vi "Syringe Freezer Interlock Configuration.vi"(8 "error in (no error)":errorcluster, 11 "cRIO-CO2 in":refnum<class "cRIO-CO2.lvclass">) -> (0 "error out":errorcluster, 2 "Interlock Chain":refnum<class "Interlock Chain.lvclass">, 3 "cRIO-CO2 out":refnum<class "cRIO-CO2.lvclass">)   [LabVIEW 2015, in "cRIO-Carbondioxide.lvlib" / "cRIO-CO2.lvlib" / "cRIO-CO2.lvclass"]
uses:
  cRIO-CO2.lvclass
  Interlocks/Interlock Chain/Interlock Chain.lvclass
  Interlocks/Interlock/Interlock.lvclass
  Interlocks/Interlock Bool/Interlock Bool.lvclass
  Interlocks/Interlock DBL/Range/Interlock Range.lvclass
  Interlocks/Interlock Bool/Interlock Bool.lvclass/Interlock Bool.ctl
  Interlocks/Interlock DBL/Range/Interlock Range.lvclass/Interlock Range.ctl
  Interlocks/Interlock Chain/Interlock Chain.lvclass/Interlock Chain.ctl
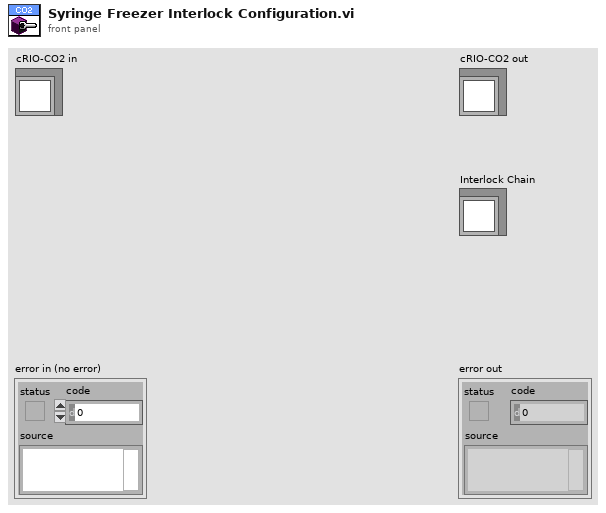
[diagram p1: front panel]
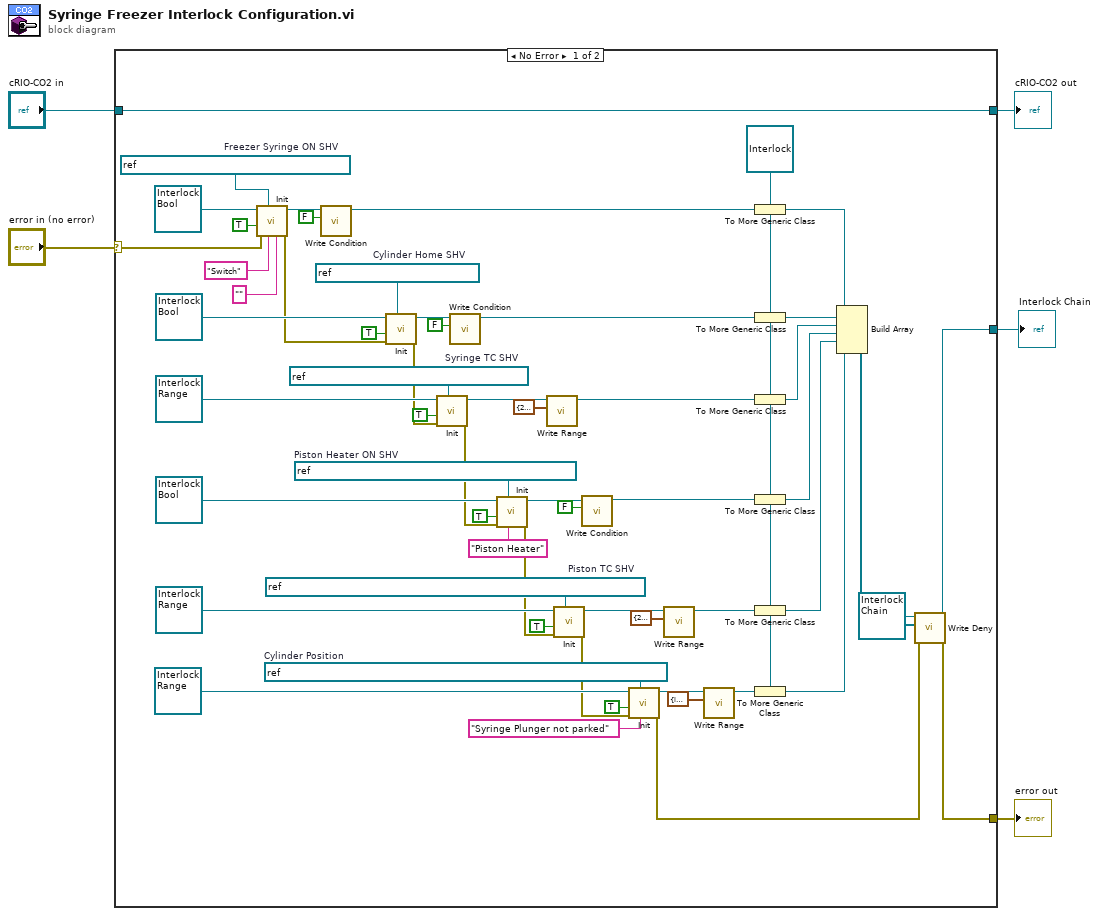
[diagram p0: block diagram]
diagram:
  n1 = case shown="No Error" "error in (no error)" {
    selector: "error in (no error)" -> [w30 w66]
    tunnel: [w25 w66] -> w4
    tunnel: [w64 w65] -> w2
    tunnel: "cRIO-CO2 in" -> [w64 w65]
    tunnel: [w22 _] -> w1
    frame No Error {
      w12 = refnum<k21> "ni.var.psp://crio-carbondioxide/AMS Gas SHV/Cylinder/Position"  # Cylinder Position
      w36 = refnum<k21> "ni.var.psp://crio-carbondioxide/AMS Gas SHV/Freezers/Freezer Syringe"  # Freezer Syringe ON SHV
      w41 = refnum<k21> "ni.var.psp://crio-carbondioxide/AMS Gas SHV/Gauges/Piston TC"  # Piston TC SHV
      w51 = refnum<k21> "ni.var.psp://crio-carbondioxide/AMS Gas SHV/Heaters/Piston Heater ON"  # Piston Heater ON SHV
      w55 = refnum<k21> "ni.var.psp://crio-carbondioxide/AMS Gas SHV/Gauges/Syringe TC"  # Syringe TC SHV
      w8 = refnum<class "Interlock.lvclass"> refnum ("Interlock.lvclass")
      w62 = refnum<k21> "ni.var.psp://crio-carbondioxide/AMS Gas SHV/Cylinder/Home"  # Cylinder Home SHV
      n2 = call-dynamic "Init.vi"("Interlock message (\" -> Interlock!\")"="" ("Interlock message (\" -> Interlock!\")"), "Name (SHV Name if empty)"="Switch", "SHV"=w36, "error in (no error)"=w30, "Stop Self on IL? (T)"=TRUE, "Interlock in"=refnum<class "Interlock Bool.lvclass"> refnum ("Interlock Bool.lvclass")) -> ("error out"=w31:errorcluster, "Interlock out"=w37:refnum<class "Interlock Bool.lvclass">)  [unwired: 4 in]
      n3 = call "Write Condition.vi"("Interlock Condition"=FALSE, "Interlock Bool in"=w37) -> ("Interlock Bool out"=w28:refnum<class "Interlock Bool.lvclass">)  [unwired: 8 in, 1 out]
      n4 = call-dynamic "Init.vi"("SHV"=w62, "error in (no error)"=w31, "Stop Self on IL? (T)"=TRUE, "Interlock in"=refnum<class "Interlock Bool.lvclass"> refnum ("Interlock Bool.lvclass")) -> ("error out"=w34:errorcluster, "Interlock out"=w61:refnum<class "Interlock Bool.lvclass">)  [unwired: 6 in]
      n5 = call-dynamic "Init.vi"("SHV"=w55, "error in (no error)"=w34, "Stop Self on IL? (T)"=TRUE, "Interlock in"=refnum<class "Interlock Range.lvclass"> refnum ("Interlock DBL.lvclass")) -> ("error out"=w33:errorcluster, "Interlock out"=w56:refnum<class "Interlock Range.lvclass">)  [unwired: 6 in]
      n6 = call "Write Condition.vi"("Interlock Condition"=FALSE, "Interlock Bool in"=w61) -> ("Interlock Bool out"=w59:refnum<class "Interlock Bool.lvclass">)  [unwired: 8 in, 1 out]
      n7 = call-dynamic "Init.vi"("Name (SHV Name if empty)"="Piston Heater", "SHV"=w51, "error in (no error)"=w33, "Stop Self on IL? (T)"=TRUE, "Interlock in"=refnum<class "Interlock Bool.lvclass"> refnum ("Interlock Bool.lvclass")) -> ("error out"=w32:errorcluster, "Interlock out"=w49:refnum<class "Interlock Bool.lvclass">)  [unwired: 5 in]
      n8 = call "Write Range.vi"("Range"=cluster{"Upper Limit":dbl, "Lower Limit":dbl} {"Upper Limit"=2000.0, "Lower Limit"=-200.0}, "Interlock Bool in"=w56) -> ("Interlock Bool out"=w53:refnum<class "Interlock Range.lvclass">)  [unwired: 8 in, 1 out]
      n9 = call-dynamic "Init.vi"("SHV"=w41, "error in (no error)"=w32, "Stop Self on IL? (T)"=TRUE, "Interlock in"=refnum<class "Interlock Range.lvclass"> refnum ("Interlock DBL.lvclass")) -> ("error out"=w15:errorcluster, "Interlock out"=w43:refnum<class "Interlock Range.lvclass">)  [unwired: 6 in]
      n10 = call "Write Condition.vi"("Interlock Condition"=FALSE, "Interlock Bool in"=w49) -> ("Interlock Bool out"=w47:refnum<class "Interlock Bool.lvclass">)  [unwired: 8 in, 1 out]
      n11 = call-dynamic "Init.vi"("Name (SHV Name if empty)"="Syringe Plunger not parked", "SHV"=w12, "error in (no error)"=w15, "Stop Self on IL? (T)"=TRUE, "Interlock in"=refnum<class "Interlock Range.lvclass"> refnum ("Interlock DBL.lvclass")) -> ("error out"=w14:errorcluster, "Interlock out"=w11:refnum<class "Interlock Range.lvclass">)  [unwired: 5 in]
      n12 = call "Write Range.vi"("Range"=cluster{"Upper Limit":dbl, "Lower Limit":dbl} {"Upper Limit"=2000.0, "Lower Limit"=20.0}, "Interlock Bool in"=w43) -> ("Interlock Bool out"=w40:refnum<class "Interlock Range.lvclass">)  [unwired: 8 in, 1 out]
      n13 = call "Write Range.vi"("Range"=cluster{"Upper Limit":dbl, "Lower Limit":dbl} {"Upper Limit"=inf, "Lower Limit"=95.0}, "Interlock Bool in"=w11) -> ("Interlock Bool out"=w9:refnum<class "Interlock Range.lvclass">)  [unwired: 8 in, 1 out]
      n14 = To More Generic Class(target class=w8, reference=w28) -> (generic class reference=w27:refnum<class "Interlock.lvclass">)
      n15 = To More Generic Class(target class=w8, reference=w59) -> (generic class reference=w58:refnum<class "Interlock.lvclass">)
      n16 = To More Generic Class(target class=w8, reference=w53) -> (generic class reference=w46:refnum<class "Interlock.lvclass">)
      n17 = To More Generic Class(target class=w8, reference=w47) -> (generic class reference=w45:refnum<class "Interlock.lvclass">)
      n18 = To More Generic Class(target class=w8, reference=w40) -> (generic class reference=w39:refnum<class "Interlock.lvclass">)
      n19 = To More Generic Class(target class=w8, reference=w9) -> (generic class reference=w7:refnum<class "Interlock.lvclass">)
      n20 = Build Array(w27, w58, w46, w45, w39, w7) -> (w23:refnum<class "Interlock.lvclass">[])
      n21 = call "Write Deny.vi"("error in (no error)"=w14, "Deny"=w23, "Interlock Chain in"=refnum<class "Interlock Chain.lvclass"> refnum) -> ("error out"=w25:errorcluster, "Interlock Chain out"=w22:refnum<class "Interlock Chain.lvclass">)  [unwired: 7 in]
    }
    frame Error {
    }
  }
  "error out" <- w4
  "cRIO-CO2 out" <- w2
  "Interlock Chain" <- w1
